vi "Programacion 1.vi"() -> ()   [LabVIEW 2011]
panel:
  out "Multiplicacion":dbl
  out "Division":dbl
  out "Resta":dbl
  out "Suma":dbl
  in  "Numeric 2":dbl
  in  "Numeric":dbl
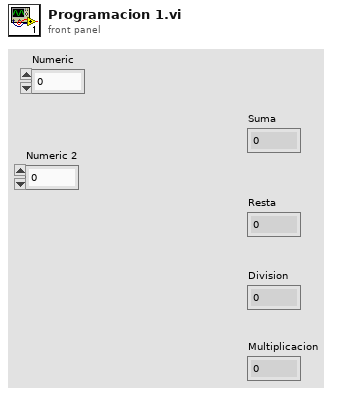
[diagram p1: front panel]
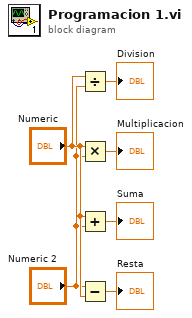
[diagram p0: block diagram]
diagram:
  n1 = Divide(x="Numeric", y="Numeric 2") -> (x/y=→"Division":dbl)
  n2 = Multiply(x="Numeric", y="Numeric 2") -> (x*y=→"Multiplicacion":dbl)
  n3 = Add(x="Numeric", y="Numeric 2") -> (x+y=→"Suma":dbl)
  n4 = Subtract(x="Numeric 2", y="Numeric") -> (x-y=→"Resta":dbl)
